vi "VisibleInvisible.vi"() -> ()   [LabVIEW 2020]
panel:
  in  "Visible":bool
  in  "stop":bool
  in  "Boolean":bool
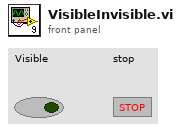
[diagram p1: front panel]
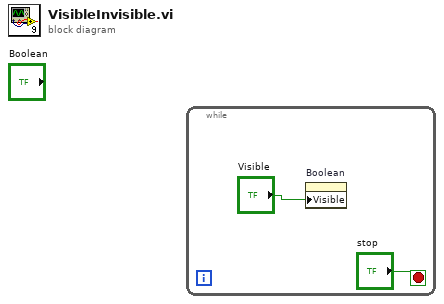
[diagram p0: block diagram]
diagram:
  n1 = while {
    stop <- "stop" stop-if-true
    n2 = property on="Boolean" class="Bool (strict)"("Visible"="Visible") -> ()  [unwired: 2 in, 2 out]
  }
